vi "Simple Analog Waveform Out.vi"() -> ()   [LabVIEW 2010]
uses:
  <vilib>/DAQmx/write.llb/DAQmx Write (Analog Wfm 1Chan NSamp).vi
  <vilib>/DAQmx/create/channels.llb/DAQmx Create Channel (AO-Voltage-Basic).vi
  <vilib>/DAQmx/configure/timing.llb/DAQmx Timing (Sample Clock).vi
  <vilib>/daqmx/miscellaneous.llb/DAQmx Fill In Error Info.vi
  <vilib>/measure/NI_MABase.lvlib
panel:
  out "number of samples written per channel":u32
  in  "# of samples":dbl
  in  "Clock & Sample Rate":dbl
  in  "x":dbl=1.64079732048 format="%#_12g"
  in  "offset":dbl=2.5
  in  "Freq (Hz)":dbl
  in  "FM Waveform Channel":tag="Dev1/ao3"
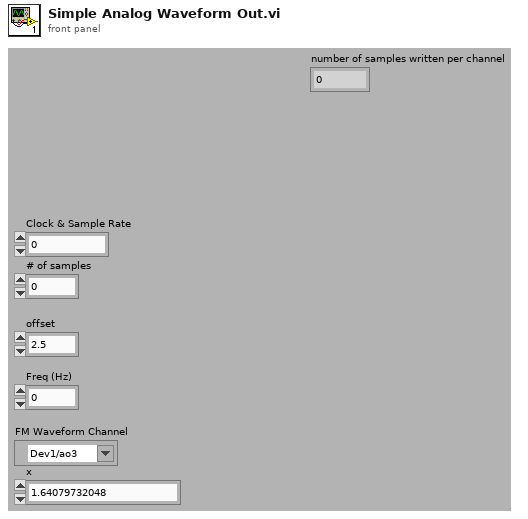
[diagram p1: front panel]
types:
  T1 = enum16{"Sine Wave", "Triangle Wave", "Square Wave", "Sawtooth Wave"}
  T2 = cluster{"Clock & Sample Rate":dbl, "# of samples":dbl}
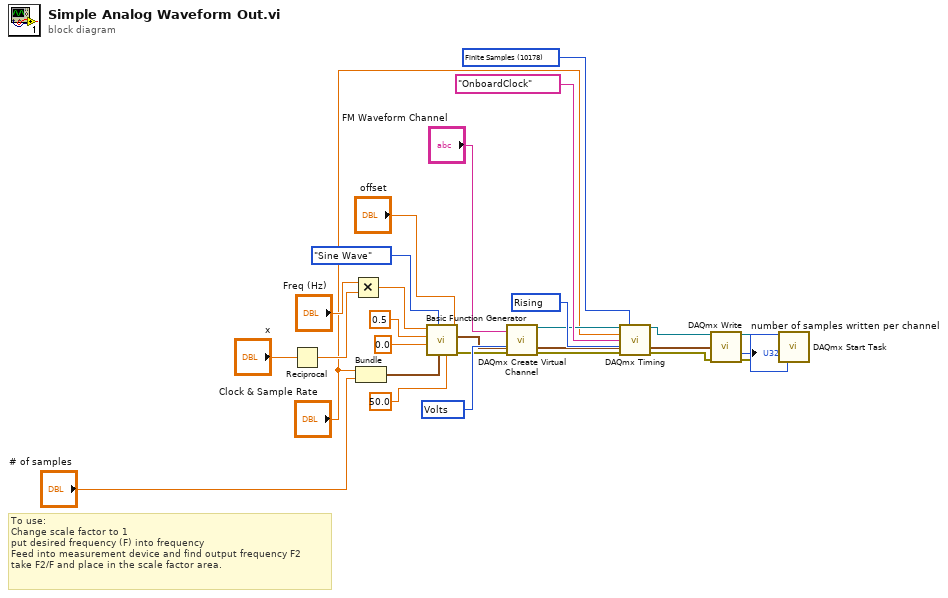
[diagram p0: block diagram]
diagram:
  w20 = 10348 items=["Volts"=10348, "From Custom Scale"=10065] ("units")
  w21 = 10178 items=["Finite Samples"=10178, "Continuous Samples"=10123, "Hardware Timed Single Point"=12522] ("sample mode")
  w22 = 10280 items=["Rising"=10280, "Falling"=10171] ("active edge")
  # "To use:\nChange scale factor to 1\nput desired frequency (F) into frequency\nFeed into measurement device and find output frequency F2\ntake F2/F and place in the scale factor area."
  n1 = Reciprocal(x="x") -> (1/x=w10:dbl)
  n2 = Multiply(x="Freq (Hz)", y=w10) -> (x*y=w11:dbl)
  n3 = Bundle("Clock & Sample Rate"="Clock & Sample Rate", "# of samples"="# of samples") -> (w8:T2)  [unwired: 1 in]
  n4 = call <vilib>:"Basic Function Generator.vi"("offset"="offset", "square wave duty cycle (%)"=50.0, "sampling info"=w8, "signal type"=T1."Sine Wave", "phase"=0.0, "amplitude"=0.5, "frequency"=w11) -> ("error out"=w16:errorcluster, "signal out"=w17:waveform(dbl))  [unwired: 2 in, 1 out]
  n5 = call-poly <vilib>:"DAQmx Create Virtual Channel.vi"("physical channels"="FM Waveform Channel", "units"=w20, "error in"=w16) -> ("task out"=w19:refnum<k21>, "error out"=w18:errorcluster)  [unwired: 11 in]
  n6 = call-poly <vilib>:"DAQmx Timing.vi"("task/channels in"=w19, "sample mode"=w21, "rate"="Clock & Sample Rate", "source"=tag "OnboardClock", "active edge"=w22, "error in"=w18) -> ("task out"=w5:refnum<k21>, "error out"=w4:errorcluster)  [unwired: 8 in]
  n7 = call-poly <vilib>:"DAQmx Write.vi"("task/channels in"=w5, "data"=w17, "error in"=w4) -> ("task out"=w3:refnum<k21>, "number of samples written per channel"=→"number of samples written per channel":u32, "error out"=w2:errorcluster)  [unwired: 10 in]
  n8 = call <vilib>:"DAQmx Start Task.vi"("task/channels in"=w3, "error in"=w2) -> ()  [unwired: 12 in, 2 out]
